vi "WT1600 Multicard Total Resistance.vi"(0 "WT1600":refnum<visa-resource-name>, 5 "error in (no error)":errorcluster) -> (14 "dup VISA session":refnum<visa-resource-name>, 15 "Total Resistance":dbl, 16 "R1":dbl, 17 "R2":dbl, 18 "R3":dbl, 19 "error out":errorcluster)   [LabVIEW 2012]
doc: "This VI only works with pattern 2. It calculates the sum of the resistance on all cards (3)"
panel:
  out "I3":dbl
  out "V3":dbl
  out "i1":dbl
  out "v1":dbl
  out "i 2":dbl
  out "v2":dbl
  out "Read Strings":string
  out "Measure":dbl[](array[numeric]) format="%^.4e"
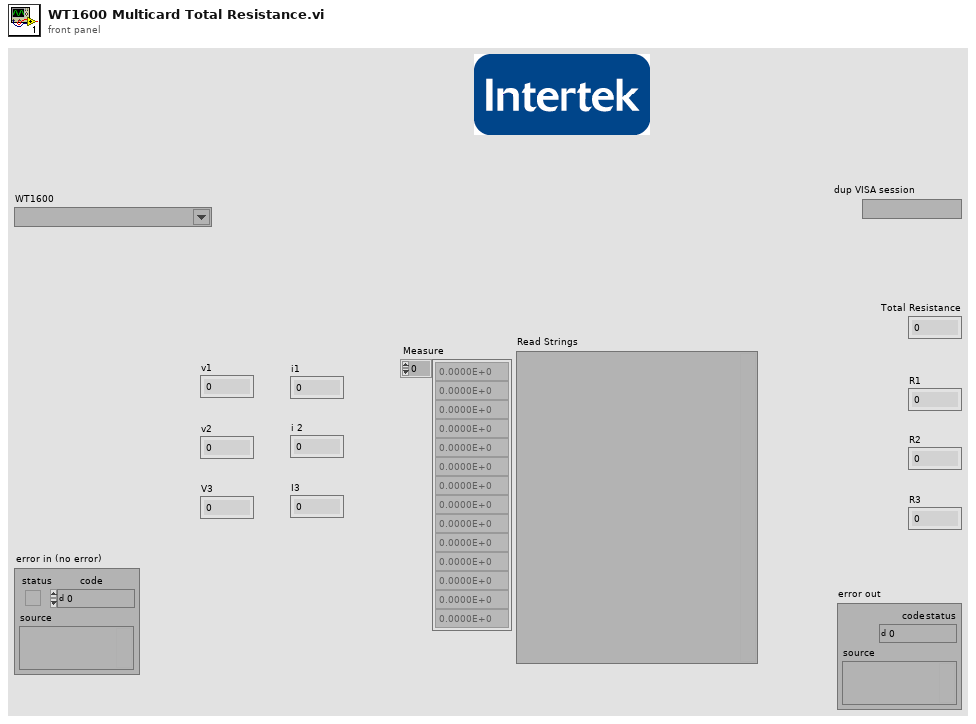
[diagram p1: front panel]
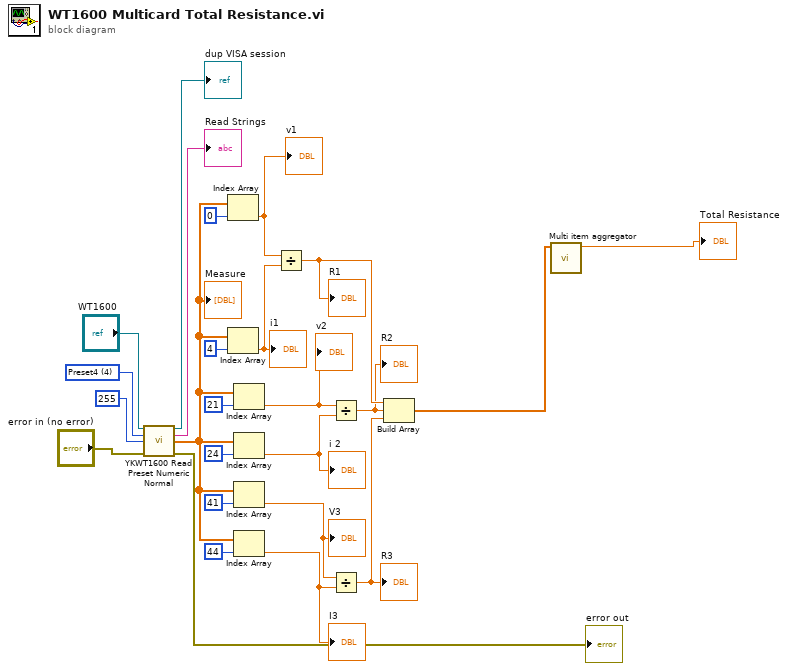
[diagram p0: block diagram]
diagram:
  w21 = u16 4 items=["", "Preset1", "Preset2", "Preset3", "Preset4"] ("Preset (2: Preset 2)")
  n1 = call <instrlib>:"YKWT1600 Read Preset Numeric Normal.vi"("VISA session"="WT1600", "Preset (2: Preset 2)"=w21, "Number of Item (15)"=u16 255, "error in (no error)"="error in (no error)") -> ("dup VISA session"=→"dup VISA session":refnum<visa-resource-name>, "Read Strings"=→"Read Strings":string, "Measure"=w18:dbl[], "error out"=→"error out":errorcluster)  [unwired: 8 in]
  "Measure" <- w18
  n2 = Index Array(array=w18, index=0) -> (element=w3:dbl)
  "v1" <- w3
  n3 = Index Array(array=w18, index=4) -> (element=w11:dbl)
  "i1" <- w11
  n4 = Index Array(array=w18, index=21) -> (element=w2:dbl)
  "v2" <- w2
  n5 = Index Array(array=w18, index=24) -> (element=w10:dbl)
  "i 2" <- w10
  n6 = Index Array(array=w18, index=41) -> (element=w1:dbl)
  "V3" <- w1
  n7 = Index Array(array=w18, index=44) -> (element=w9:dbl)
  "I3" <- w9
  n8 = Divide(x=w3, y=w11) -> (x/y=w8:dbl)
  "R1" <- w8
  n9 = Divide(x=w2, y=w10) -> (x/y=w7:dbl)
  "R2" <- w7
  n10 = Divide(x=w1, y=w9) -> (x/y=w6:dbl)
  "R3" <- w6
  n11 = Build Array(w8, w7, w6) -> (w5:dbl[])
  n12 = call "Multi item aggregator.vi"("Array"=w5) -> ("Numeric"=→"Total Resistance":dbl)  [unwired: 10 in]
